vi "Untitled 1.vi"() -> ()   [LabVIEW 2021]
panel:
  out "String 2":string
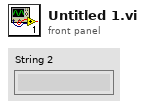
[diagram p1: front panel]
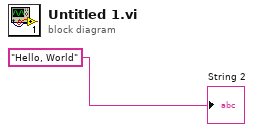
[diagram p0: block diagram]
diagram:
  "String 2" <- "Hello, World" ("String")
